vi "FFT.vi"(8 "error in (no error)":errorcluster, 11 "FFT in":refnum<class "FFT.lvclass">) -> (0 "error out":errorcluster, 3 "FFT out":refnum<class "FFT.lvclass">)   [LabVIEW 2014, in "AnalysisPlugins.lvlib" / "FFT.lvclass"]
uses:
  FFT.lvclass
  AnalysisPluginBaseClass/AnalysisPluginsBase.lvclass/AnalysisPluginsBase.ctl
  FFT.lvclass/FFT.ctl
  Typedefs/FftReport.ctl
  AnalysisPluginBaseClass/Accessors/Write Result.vi
  AnalysisPluginBaseClass/Accessors/Read Window.vi
  Accessors/Read WindowFunction.vi
  Accessors/Read FftView.vi
  <vilib>/measure/maspectr.llb/FFT Spectrum (Mag-Phase) for 1 Chan.vi
  <vilib>/measure/NI_MAPro.lvlib
panel:
  out "DFT":waveform(dbl)[](graph)
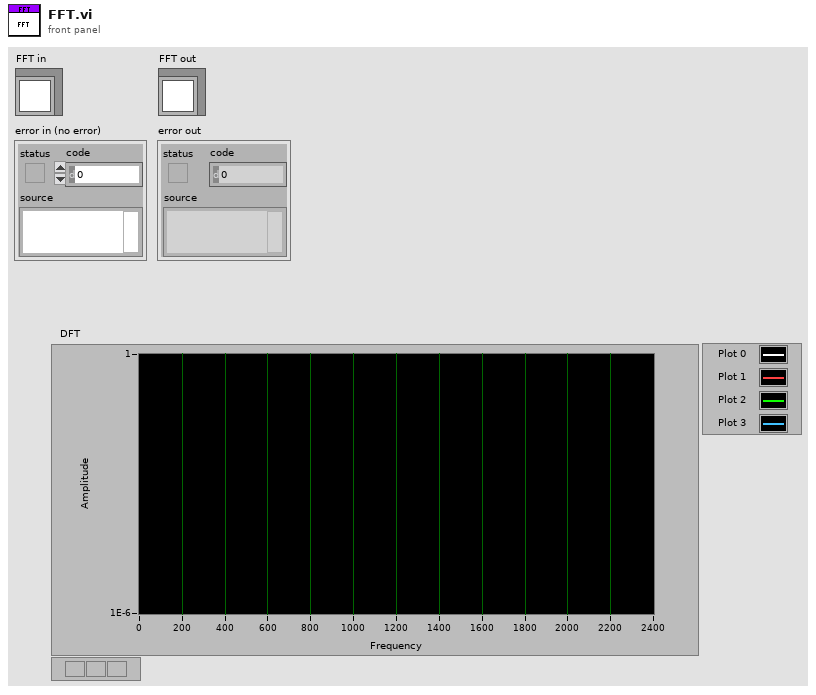
[diagram p1: front panel]
types:
  T1 = typedef "AnalysisPlugins.lvlib/FFT.lvclass/FftReport.ctl" = cluster{"dF":dbl, "FFT":cdb[][], "F0":dbl}
  T2 = typedef "AnalysisPlugins.lvlib/AnalysisPluginsBase.lvclass/clWindowData.ctl" = cluster{"Timestamp":ext, "Samples":dbl[][], "Window Valid":bool}
  T3 = typedef "AnalysisPlugins.lvlib/FitterBase.lvclass/clAnalysisConfig.ctl" = cluster{"F0":u32, "SettlingTime":dbl, "AnalysisCycles":dbl, "SampleRate":dbl, "NumChannels":u32, "TsOffset":enum16{"start", "middle", "end"}}
  T4 = typedef "NI_AALPro.lvlib/windowTd.ctl" = u32
  T5 = typedef "AnalysisPlugins.lvlib/FFT.lvclass/FftView2.ctl" = cluster{"dB On (F)":bool, "unwrap phase (F)":bool, "convert to degree (F)":bool}
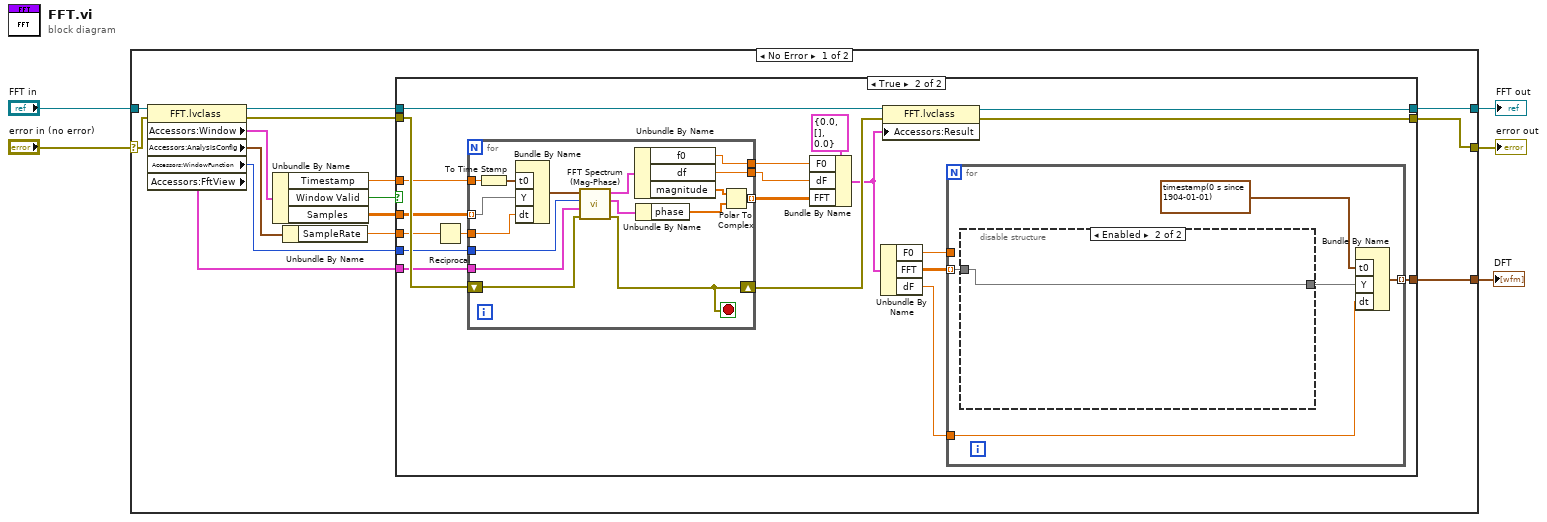
[diagram p0: block diagram]
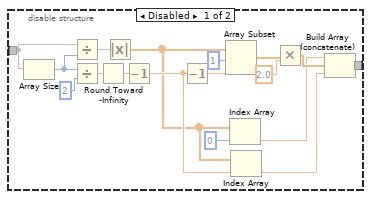
[diagram p3: hidden frame]
diagram:
  n1 = case shown="No Error" "error in (no error)" {
    selector: "error in (no error)" -> [w19 w83]
    tunnel: [w9 w83] -> w4
    tunnel: [w15 w82] -> w2
    tunnel: "FFT in" -> [w20 w82]
    tunnel: [w8 _] -> w1
    frame No Error {
      n2 = property class="FFT.lvclass"(reference=w20, error in=w19) -> (reference out=w16:refnum<class "FFT.lvclass">, error out=w13:errorcluster, "Accessors:Window"=w17:T2, "Accessors:AnalysisConfig"=w18:T3, "Accessors:WindowFunction"=w7:T4, "Accessors:FftView"=w6:T5)
      n3 = Unbundle By Name(w17) -> ("Timestamp"=w10:ext, "Window Valid"=w14:bool, "Samples"=w12:dbl[][])
      n4 = Unbundle By Name(w18) -> ("SampleRate"=w11:dbl)
      n5 = case shown="True" w14 {
        tunnel: w16 -> [w22 w40]
        tunnel: [w22 w38] -> w15
        tunnel: w13 -> [w21 w42]
        tunnel: w12 -> [_ w29]
        tunnel: w11 -> [_ w30]
        tunnel: w10 -> [_ w41]
        tunnel: [w21 w37] -> w9
        tunnel: [_ w36] -> w8
        tunnel: w7 -> [_ w28]
        tunnel: w6 -> [_ w27]
        frame False {
        }
        frame True {
          n6 = Reciprocal(x=w30) -> (1/x=w23:dbl)
          n7 = for {
            tunnel: w41 -> [w58]
            tunnel: w29 -> [w56] mode=indexing
            tunnel: w23 -> [w55]
            tunnel: w28 -> [w53]
            tunnel: w27 -> [w52]
            tunnel: [w46] -> w24 mode=indexing
            tunnel: [w45] -> w26
            tunnel: [w44] -> w25
            shift-right: [w43] -> w39
            shift-left: w42 -> [w51]
            stop <- w43 stop-if-true
            n8 = To Time Stamp(1:w58) -> (0:w57:timestamp)
            n9 = Bundle By Name("t0"=w57, "Y"=w56, "dt"=w55) -> (w54:waveform(dbl))  [unwired: 1 in]
            n10 = call-poly <vilib>:"FFT Spectrum (Mag-Phase).vi"("error in (no error)"=w51, "view"=w52, "window"=w53, "time signal"=w54) -> ("error out"=w43:errorcluster, "phase"=w49:cluster{"f0":dbl, "df":dbl, "phase":dbl[]}, "magnitude"=w50:cluster{"f0":dbl, "df":dbl, "magnitude":dbl[]})  [unwired: 3 in, 2 out]
            n11 = Unbundle By Name(w50) -> ("f0"=w44:dbl, "df"=w45:dbl, "magnitude"=w48:dbl[])
            n12 = Unbundle By Name(w49) -> ("phase"=w47:dbl[])
            n13 = Polar To Complex(1:w47, 2:w48) -> (0:w46:cdb[])
          }
          n14 = Bundle By Name(cluster=T1 {"dF"=0.0, "FFT"=[], "F0"=0.0} ("FftReport"), "F0"=w25, "dF"=w26, "FFT"=w24) -> (w34:T1)
          n15 = Unbundle By Name(w34) -> ("F0"=w33:dbl, "FFT"=w32:cdb[][], "dF"=w31:dbl)
          n16 = property class="FFT.lvclass"(reference=w40, error in=w39, "Accessors:Result"=w34) -> (reference out=w38:refnum<class "FFT.lvclass">, error out=w37:errorcluster)
          n17 = for {
            tunnel: [w62] -> w36 mode=indexing
            tunnel: w33 -> [_]
            tunnel: w32 -> [w60] mode=indexing
            tunnel: w31 -> [w61]
            n18 = disable-structure shown="Enabled" {
              disable-tunnel: w60 -> [w77 w81]
              disable-tunnel: [w73 w81] -> w59
              frame Disabled {
                n19 = Array Size(array=w77) -> (size(s)=w76:i32)
                n20 = Divide(x=w77, y=w76) -> (x/y=w80:cdb[])
                n21 = Divide(x=w76, y=2) -> (x/y=w79:dbl)
                n22 = Round Toward -Infinity(1:w79) -> (0:w67:dbl)
                n23 = Absolute Value(x=w80) -> (abs(x)=w64:dbl[])
                n24 = Decrement(x=w67) -> (x-1=w65:dbl)
                n25 = Decrement(x=w65) -> (x-1=w66:dbl)
                n26 = Array Subset(array=w64, index=1, length=w66) -> (w71:dbl[])
                n27 = Index Array(array=w64, index=0) -> (element=w74:dbl)
                n28 = Index Array(array=w64, index=w65) -> (element=w68:dbl)
                n29 = Multiply(x=w71, y=2.0) -> (x*y=w75:dbl[])
                n30 = Build Array (concatenate)(w74, w75, w68) -> (w73:dbl[])
              }
              frame Enabled {
              }
            }
            n31 = Bundle By Name("t0"=timestamp(0 s since 1904-01-01), "Y"=w59, "dt"=w61) -> (w62:waveform(cdb))  [unwired: 1 in]
          }
        }
      }
    }
    frame Error {
    }
  }
  "error out" <- w4
  "FFT out" <- w2
  "DFT" <- w1
